vi "Parse Hand.vi"(7 "Hand History String":string, 9 "Card Map In":T2(array[cluster]), 10 "Chip Stacks":dbl[][](array[numeric]), 11 "Player Names":string[](array[string])) -> (1 "Card Map Out":T1(array[cluster]), 2 "Chip Stacks Out":dbl[][](array[numeric]), 3 "Player Names Out":string[](array[string]))   [LabVIEW 2021]
uses:
  15104598-1371-43f4-918d-030f7d83b414.vi
  <vilib>/Comparison/Equal/Equal Functor/Equal Functor.lvclass
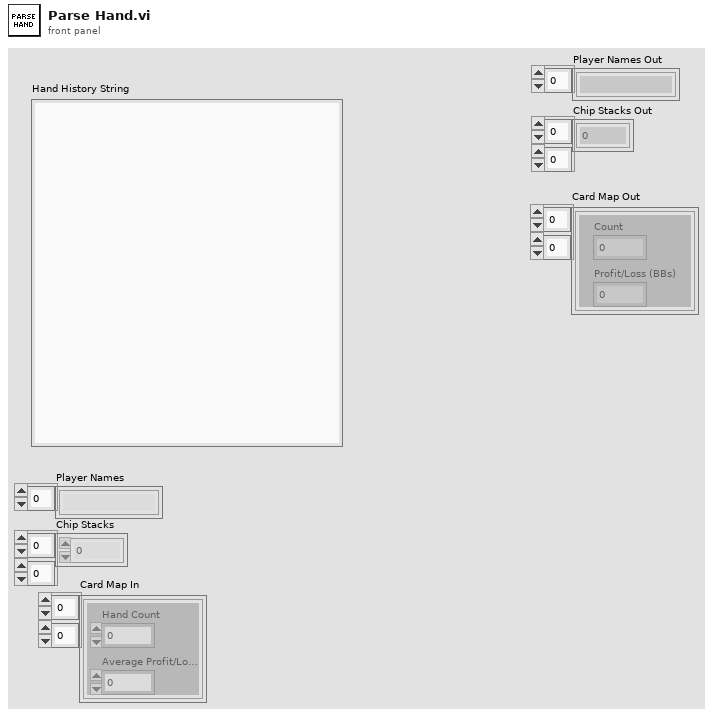
[diagram p1: front panel]
types:
  T1 = cluster{"Count":u16, "Profit/Loss (BBs)":dbl}[][]
  T2 = cluster{"Hand Count":u16, "Average Profit/Loss (BBs)":dbl}[][]
  T3 = cluster{"Hand Count":u16, "Average Profit/Loss (BBs)":dbl}
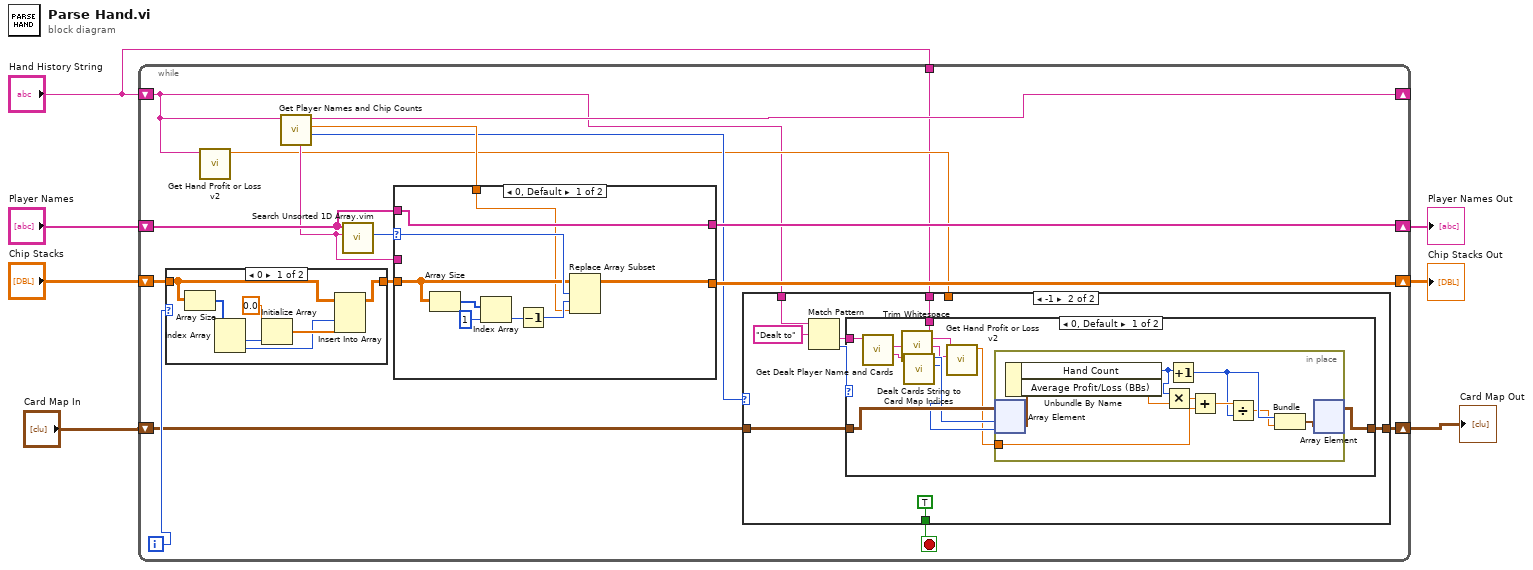
[diagram p0: block diagram]
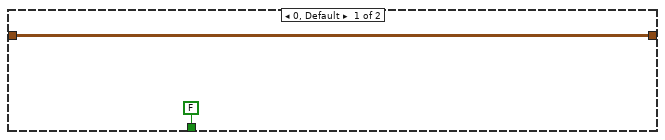
[diagram p2: hidden frame]
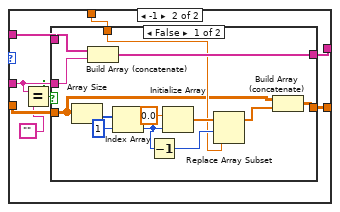
[diagram p5: hidden frame]
diagram:
  n1 = while {
    shift-right: [w21] -> w5
    shift-left: "Player Names" -> [w23]
    shift-right: [w19] -> w4
    shift-left: "Chip Stacks" -> [w18]
    shift-right: [w11] -> _
    shift-left: "Hand History String" -> [w9]
    shift-right: [w13] -> w2
    shift-left: "Card Map In" -> [w12]
    tunnel: "Hand History String" -> [w8]
    i -> [w16]
    stop <- w14 stop-if-true
    n2 = case shown="0" w16 {
      tunnel: w18 -> [w58 w62]
      tunnel: [w57 w62] -> w17
      frame 0 {
        n3 = Array Size(array=w58) -> (size(s)=w61:i32[])
        n4 = Index Array(array=w61) -> (element #1=w60:i32, element #2=w55:i32)  [unwired: 2 in]
        n5 = Initialize Array(0.0 ("element"), w60) -> (w56:dbl[])
        n6 = Insert Into Array(array=w58, index (col)=w55, new element=w56) -> (w57:dbl[][])  [unwired: 1 in]
      }
      frame 1, Default {
      }
    }
    n7 = call "Get Hand Profit or Loss v2.vi"("Hand History String"=w9) -> ("Profit/Loss (BBs)"=w10:dbl)  [unwired: 10 in]
    n8 = call "Get Player Names and Chip Counts.vi"("Hand History String in"=w9) -> ("End of players = -1"=w15:i32, "Chip Count"=w20:dbl, "Hand History String out"=w11:string, "Player"=w22:string)  [unwired: 7 in]
    n9 = call "Search Unsorted 1D Array.vim"("element"=w22, "unsorted 1D array"=w23) -> ("index of element"=w24:i32)  [unwired: 9 in]
    n10 = case shown="0, Default" w24 {
      selector: w24 -> [w70 _]
      tunnel: w17 -> [w69 w76]
      tunnel: w23 -> [w71 w79]
      tunnel: w22 -> [_ w74]
      tunnel: [w71 w78] -> w21
      tunnel: w20 -> [w64 w77]
      tunnel: [w63 w75] -> w19
      frame 0, Default {
        n11 = Array Size(array=w69) -> (size(s)=w68:i32[])
        n12 = Index Array(array=w68, index=1) -> (element=w66:i32)
        n13 = Decrement(x=w66) -> (x-1=w65:i32)
        n14 = Replace Array Subset(array=w69, new element=w64, index (row)=w70, index (col)=w65) -> (w63:dbl[][])
      }
      frame -1 {
        n15 = Equal?(x=w74, y="") -> (x = y?=w72:bool)
        n16 = case shown="False" w72 {
          tunnel: w79 -> [w92 w94]
          tunnel: w74 -> [w91 _]
          tunnel: [w90 w94] -> w78
          tunnel: w77 -> [w83 _]
          tunnel: w76 -> [w82 w93]
          tunnel: [w81 w93] -> w75
          frame False {
            n17 = Array Size(array=w82) -> (size(s)=w89:i32[])
            n18 = Build Array (concatenate)(w92, w91) -> (w90:string[])
            n19 = Index Array(array=w89, index=1) -> (element=w85:i32)
            n20 = Decrement(x=w85) -> (x-1=w84:i32)
            n21 = Initialize Array(0.0 ("element"), w85) -> (w86:dbl[])
            n22 = Replace Array Subset(array=w86, new element=w83, index=w84) -> (w80:dbl[])
            n23 = Build Array (concatenate)(w82, w80) -> (w81:dbl[][])
          }
          frame True {
          }
        }
      }
    }
    n24 = case shown="-1" w15 {
      tunnel: [FALSE TRUE] -> w14
      tunnel: w9 -> [_ w28]
      tunnel: [w25 w29] -> w13
      tunnel: w12 -> [w25 w30]
      tunnel: w10 -> [_ _]
      tunnel: w8 -> [_ w27]
      frame 0, Default {
      }
      frame -1 {
        n25 = Match Pattern(string=w28, regular expression="Dealt to") -> (after substring=w32:string, offset past match=w31:i32)  [unwired: 1 in, 2 out]
        n26 = case shown="0, Default" w31 {
          tunnel: w32 -> [w44 _]
          tunnel: w30 -> [w40 w54]
          tunnel: [w37 w54] -> w29
          tunnel: w27 -> [w41 _]
          frame 0, Default {
            n27 = call "Get Dealt Player Name and Cards.vi"("Hand History String in"=w44) -> ("Dealt Cards"=w43:string, "Dealt Player Name"=w42:string)  [unwired: 8 in, 1 out]
            n28 = call <vilib>:"Trim Whitespace.vi"("string"=w42) -> ("trimmed string"=w35:string)  [unwired: 1 in]
            n29 = call "Dealt Cards String to Card Map Indices.vi"("Dealt Cards String"=w43) -> ("Index1"=w38:i32, "Index0"=w39:i32)  [unwired: 9 in]
            n30 = call "Get Hand Profit or Loss v2.vi"("Dealt Player Name"=w35, "Hand History String"=w41) -> ("Profit/Loss (BBs)"=w36:dbl)  [unwired: 9 in]
            n31 = in-place {
              in-place-border: w36 -> [w48]
              n32 = in-place-array #1(w40, w39, w38) -> (w53:T3)
              n33 = Unbundle By Name(w53) -> ("Hand Count"=w50:u16, "Average Profit/Loss (BBs)"=w51:dbl)
              n34 = Multiply(x=w50, y=w51) -> (x*y=w49:dbl)
              n35 = Increment(x=w50) -> (x+1=w46:u16)
              n36 = Add(x=w49, y=w48) -> (x+y=w47:dbl)
              n37 = Divide(x=w47, y=w46) -> (x/y=w45:dbl)
              n38 = Bundle(w46, w45) -> (w52:cluster{u16, dbl})  [unwired: 1 in]
              n39 = in-place-array #1(w52) -> (w37:T2)  [unwired: 2 out]
            }
          }
          frame -1 {
          }
        }
      }
    }
  }
  "Player Names Out" <- w5
  "Chip Stacks Out" <- w4
  "Card Map Out" <- w2
